vi "GUI.vi"(8 "error in":errorcluster, 11 "Oscilloscope in":refnum<class "Oscilloscope.lvclass">) -> (0 "error out":errorcluster, 3 "Oscilloscope out":refnum<class "Oscilloscope.lvclass">)   [LabVIEW 2019, in "Oscilloscope.lvlib" / "Oscilloscope.lvclass"]
uses:
  Oscilloscope.lvclass
  Custom Controls/Horizontal Setting.ctl
  Custom Controls/Trigger Settings.ctl
  Custom Controls/Edge Select.ctl
  Custom Controls/Channel List.ctl
  Custom Controls/Trigger Coupling.ctl
  Custom Controls/Trigger Modifier.ctl
  Custom Controls/Trigger Type.ctl
  C:/Users/Public/Documents/Development/builds/Instruments/Instruments.lvlibp/Library/Instruments.lvclass
  Custom Controls/Channel Settings.ctl
  Custom Controls/Vertical Coupling.ctl
  Oscilloscope.lvclass/Oscilloscope.ctl
  Accessors/Write Horizontal Setting.vi
  Accessors/Write Trigger Settings.vi
  Accessors/Read Trigger Settings.vi
  Accessors/Read Horizontal Setting.vi
  builds/Instruments/Instruments.lvlibp/Accessors/Read dt.vi
  Accessors/Read Channel Setting.vi
  Accessors/Write Channel Setting.vi
panel:
  in  "Channel List":T1 items=["Channel_1", "Channel_2", "Channel_3", "Channel_4", "Channel_5", "Channel_6", "Channel_7", "Channel_8"]
  in  "Channel Settings":T2={"Amplitude"=0.0, "Vertical Coupling"=enum."DC", "Probe Attenuation"=1.0, "Enable?"=FALSE, "Maximum Input Frequency"=0.0, "Input Impedance"=0, "Timeout (s)"=5.0} {"Timeout (s)" format="%.2f"; "Input Impedance" items=["1 mega ohm", "50 ohms"]; "Maximum Input Frequency" format="%.2f"}
  in  "stop":bool
  in  "Trigger Settings":T4={"Edge:"=0, "Level"=0.0, "Source"=0, "trigger coupling"=1, "Holdoff"=0.0, "Delay"=0.0, "Trigger Modifier"=enum."Auto Trigger", "Trigger Type"=enum."Analog Edge"} {"Delay" format="%_6g"; "Level" format="%_6g"; "Edge:" items=["Rising Edge", "Falling Edge"]; "Holdoff" format="%_6g"; "trigger coupling" items=["AC", "DC", "HF Reject", "LF Reject", "AC Plus HF Reject"]; "Source" items=["Channel_1", "Channel_2", "Channel_3", "Channel_4", "Channel_5", "Channel_6", "Channel_7", "Channel_8"]}
  out "Waveform Graph":waveform(dbl)[](graph)
  in  "Horizontal Setting":T9={"Num Records"=0, "Sample Rate"=915.5, "Reference Pos"=50.0, "Min Record len"=1000} caption="Horizontal"
  # "Oscilloscope:"
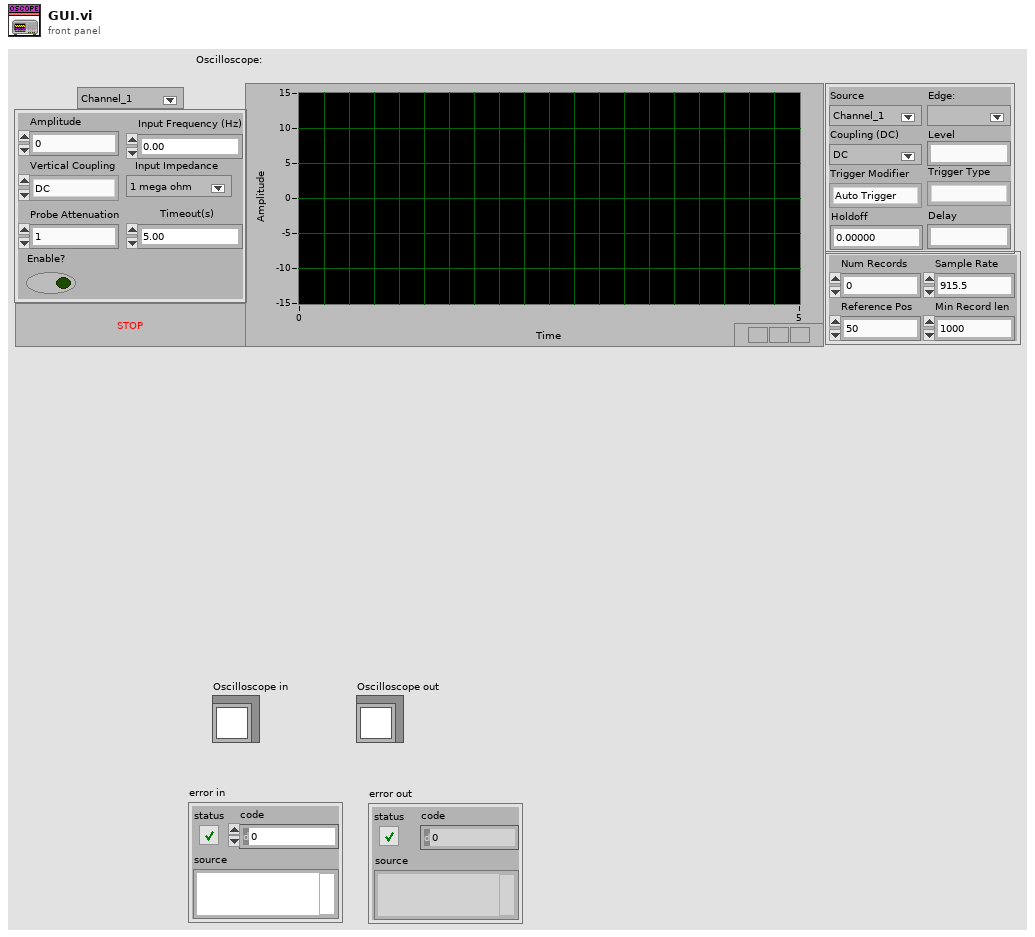
[diagram p1: front panel]
types:
  T1 = typedef "Oscilloscope.lvlib/Oscilloscope.lvclass/Channel List.ctl" = u16
  T2 = typedef "Oscilloscope.lvlib/Oscilloscope.lvclass/Channel Settings.ctl" = cluster{"Amplitude":dbl, "Vertical Coupling":T3, "Probe Attenuation":dbl, "Enable?":bool, "Maximum Input Frequency":dbl, "Input Impedance":u16, "Timeout (s)":dbl}
  T3 = typedef "Oscilloscope.lvlib/Oscilloscope.lvclass/Vertical Coupling.ctl" = enum16{"AC", "DC", "Ground"}
  T4 = typedef "Oscilloscope.lvlib/Oscilloscope.lvclass/Trigger Settings.ctl" = cluster{"Edge:":T5, "Level":dbl, "Source":T1, "trigger coupling":T6, "Holdoff":dbl, "Delay":dbl, "Trigger Modifier":T7, "Trigger Type":T8}
  T5 = typedef "Oscilloscope.lvlib/Oscilloscope.lvclass/Edge Select.ctl" = u16
  T6 = typedef "Oscilloscope.lvlib/Oscilloscope.lvclass/Trigger Coupling.ctl" = u16
  T7 = typedef "Oscilloscope.lvlib/Oscilloscope.lvclass/Trigger Modifier.ctl" = enum16{"Invalid_Setting", "None", "Auto Trigger"}
  T8 = typedef "Oscilloscope.lvlib/Oscilloscope.lvclass/Trigger Type.ctl" = enum16{"Immediate", "Analog Edge", "Digital", "Window", "Hysteresis"}
  T9 = typedef "Oscilloscope.lvlib/Oscilloscope.lvclass/Horizontal Setting.ctl" = cluster{"Num Records":i32, "Sample Rate":dbl, "Reference Pos":dbl, "Min Record len":i32}
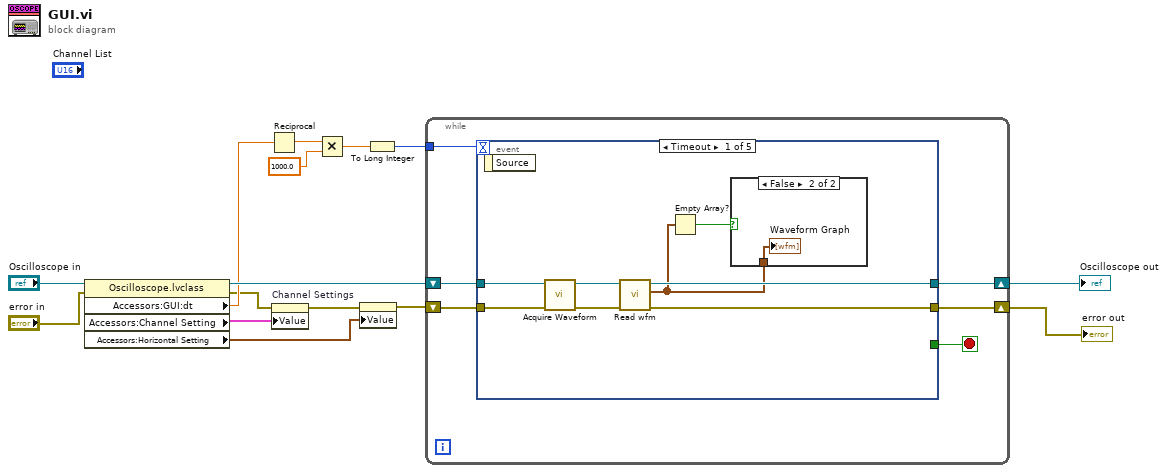
[diagram p0: block diagram]
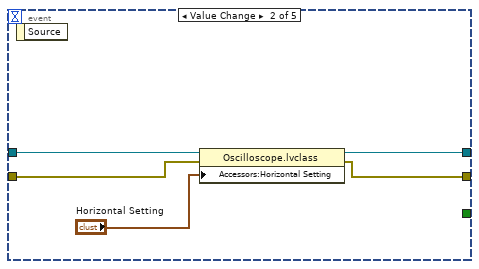
[diagram p3: hidden frame]
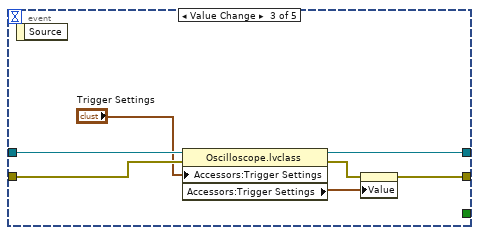
[diagram p4: hidden frame]
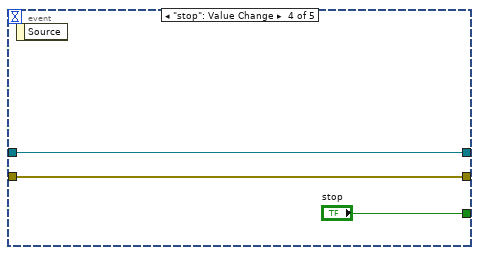
[diagram p5: hidden frame]
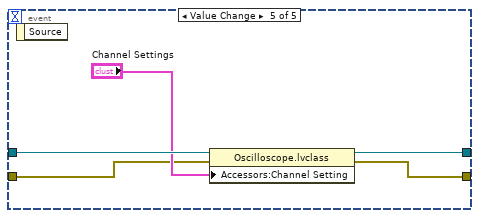
[diagram p6: hidden frame]
diagram:
  n1 = property class="Oscilloscope.lvclass"(reference="Oscilloscope in", error in="error in") -> (reference out=w10:refnum<class "Oscilloscope.lvclass">, error out=w2:errorcluster, "Accessors:GUI:dt"=w8:dbl, "Accessors:Channel Setting"=w1:T2, "Accessors:Horizontal Setting"=w9:T9)
  n2 = Reciprocal(x=w8) -> (1/x=w7:dbl)
  n3 = property on="Channel Settings" class="Clust (strict)"(error in=w2, "Value"=w1) -> (error out=w3:errorcluster)  [unwired: 1 in, 1 out]
  n4 = Multiply(x=w7, y=1000.0) -> (x*y=w5:dbl)
  n5 = property on="Horizontal Setting" class="Clust (strict)"(error in=w3, "Value"=w9) -> (error out=w15:errorcluster)  [unwired: 1 in, 1 out]
  n6 = To Long Integer(number=w5) -> (32bit integer=w4:i32)
  n7 = while {
    shift-right: [w20] -> w14
    shift-left: w10 -> [w21]
    shift-right: [w18] -> w13
    shift-left: w15 -> [w19]
    tunnel: w4 -> [w16]
    stop <- w17 stop-if-true
    n8 = event shown="[0] Timeout" {
      selector: _ -> [_ _ _ _ _]
      dyn-events: _ -> [_ _ _ _ _]
      timeout: w16 -> [_ _ _ _ _]
      tunnel: w21 -> [w26 w35 w42 w45 w50]
      tunnel: [w28 w34 w41 w45 w49] -> w20
      tunnel: [w29 w31 w36 w44 w46] -> w18
      tunnel: w19 -> [w27 w32 w40 w44 w47]
      tunnel: [_ _ _ "stop" _] -> w17
      event Timeout {
        n9 = event-data() -> ()  [unwired: 1 in, 1 out]
        n10 = call-dynamic "Acquire Waveform.vi"("error in (no error)"=w27, "Oscilloscope in"=w26) -> ("error out"=w25:errorcluster, "Oscilloscope out"=w24:refnum<class "Oscilloscope.lvclass">)  [unwired: 7 in, 1 out]
        n11 = call "Read wfm.vi"("error in (no error)"=w25, "Oscilloscope in"=w24) -> ("error out"=w29:errorcluster, "wfm"=w23:waveform(dbl)[], "Oscilloscope out"=w28:refnum<class "Oscilloscope.lvclass">)  [unwired: 7 in]
        n12 = Empty Array?(array=w23) -> (empty?=w22:bool)
        n13 = case shown="False" w22 {
          tunnel: w23 -> [_ w30]
          frame True {
          }
          frame False {
            "Waveform Graph" <- w30
          }
        }
      }
      event Value Change {
        n14 = event-data() -> ()  [unwired: 1 in, 1 out]
        n15 = property class="Oscilloscope.lvclass"(reference=w35, error in=w32, "Accessors:Horizontal Setting"="Horizontal Setting") -> (reference out=w34:refnum<class "Oscilloscope.lvclass">, error out=w31:errorcluster)
      }
      event Value Change {
        n16 = event-data() -> ()  [unwired: 1 in, 1 out]
        n17 = property class="Oscilloscope.lvclass"(reference=w42, error in=w40, "Accessors:Trigger Settings"="Trigger Settings") -> (reference out=w41:refnum<class "Oscilloscope.lvclass">, error out=w37:errorcluster, "Accessors:Trigger Settings"=w38:T4)
        n18 = property on="Trigger Settings" class="Clust (strict)"(error in=w37, "Value"=w38) -> (error out=w36:errorcluster)  [unwired: 1 in, 1 out]
      }
      event "stop": Value Change {
        n19 = event-data() -> ()  [unwired: 1 in, 1 out]
      }
      event Value Change {
        n20 = event-data() -> ()  [unwired: 1 in, 1 out]
        n21 = property class="Oscilloscope.lvclass"(reference=w50, error in=w47, "Accessors:Channel Setting"="Channel Settings") -> (reference out=w49:refnum<class "Oscilloscope.lvclass">, error out=w46:errorcluster)
      }
    }
  }
  "Oscilloscope out" <- w14
  "error out" <- w13
